vi "url to meter reading.vi"(7 "Meter1":string, 8 "Error In":errorcluster) -> (0 "error out":errorcluster, 2 "to indicator":dbl, 3 "to spreadsheet":dbl, 4 "is zero?":bool)   [LabVIEW 2015]
panel:
  out "length":i32
  out "String":string
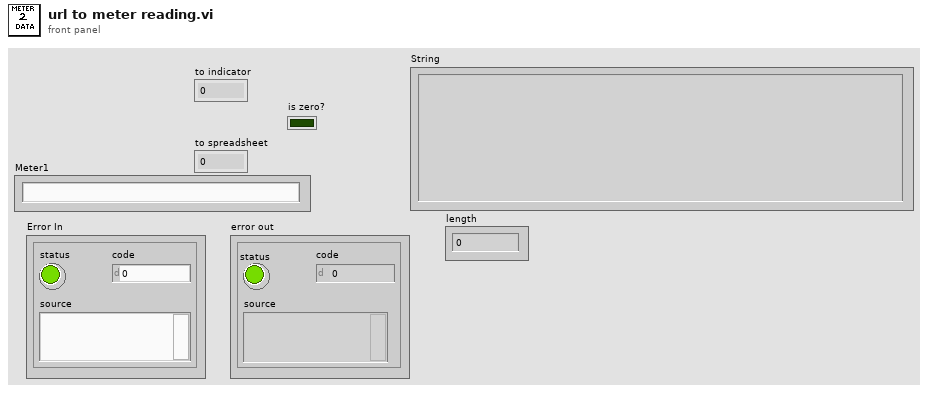
[diagram p1: front panel]
types:
  T1 = enum16{"Read", "Write", "ReadWrite", "BufferedRead", "BufferedReadWrite"}
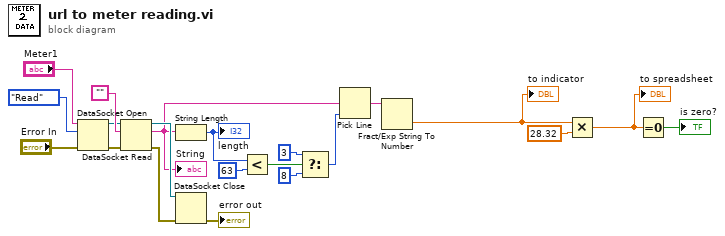
[diagram p0: block diagram]
diagram:
  n1 = DataSocket Open(8:"Error In", 10:T1."Read", 11:"Meter1") -> (0:w19:errorcluster, 3:w12:refnum<k13>)  [unwired: 1 in]
  n2 = DataSocket Read(8:w19, 10:"", 11:w12) -> (0:w18:errorcluster, 2:w3:string, 3:w11:refnum<k13>)  [unwired: 2 in, 4 out]
  "String" <- w3
  n3 = String Length(string=w3) -> (length=w5:i32)
  "length" <- w5
  n4 = DataSocket Close(8:w18, 11:w11) -> (0:→"error out":errorcluster)  [unwired: 1 in, 1 out]
  n5 = Less?(x=w5, y=63) -> (x < y?=w4:bool)
  n6 = Select(t=3, s=w4, f=8) -> (s? t:f=w2:i32)
  n7 = Pick Line(multi-line string=w3, line index=w2) -> (output string=w1:string)  [unwired: 1 in]
  n8 = Fract/Exp String To Number(string=w1) -> (number=w14:dbl)  [unwired: 3 in, 1 out]
  "to indicator" <- w14
  n9 = Multiply(x=w14, y=28.32) -> (x*y=w13:dbl)
  "to spreadsheet" <- w13
  n10 = Equal To 0?(x=w13) -> (x = 0?=→"is zero?":bool)
